vi "231124_Nikon_Led.vi"(8 "error in":errorcluster, 10 "Light path":u16(ring) items=["1- Eyepiece"=1, "2- Right"=2, "3- Left + Eyepiece"=3, "4- Left"=4], 11 "Microscope IN":T1={"Init"=FALSE, "ON / OFF"=FALSE, "Intensity"=102.0, "Objective"=2, "Light path"=1, "Z pos (µm)"=48440, "Eyepiece"=FALSE, "Right"=FALSE, "Left + Eyepiece"=FALSE, "Left"=FALSE} {"Z pos (µm)" min=0 max=990000 step=100 scale=0.0..990000.0; "Light path" items=["1- Eyepiece"=1, "2- Right"=2, "3- Left + Eyepiece"=3, "4- Left"=4]; "Objective" items=["1- Target"=1, "2- PLAN APO 100X 1,45 Oil"=2, "3- Empty"=3, "4- Empty"=4, "5- Empty"=5, "6- Empty"=6]; "Intensity" scale=0.0..2100.0}) -> (0 "error out":errorcluster, 3 "Microscope OUT":T1={"Init"=FALSE, "ON / OFF"=FALSE, "Intensity"=102.0, "Objective"=2, "Light path"=1, "Z pos (µm)"=48440, "Eyepiece"=FALSE, "Right"=FALSE, "Left + Eyepiece"=FALSE, "Left"=FALSE} {"Z pos (µm)" min=0 max=990000 step=100 scale=0.0..990000.0; "Light path" items=["1- Eyepiece"=1, "2- Right"=2, "3- Left + Eyepiece"=3, "4- Left"=4]; "Objective" items=["1- Target"=1, "2- PLAN APO 100X 1,45 Oil"=2, "3- Empty"=3, "4- Empty"=4, "5- Empty"=5, "6- Empty"=6]; "Intensity" scale=0.0..2100.0})   [LabVIEW 2024]
doc: "Thi vi displays LEDs accordingly to the lightpath"
panel:
  # "White light"
  # "Objective"
  # "Light path"
  # "Z pos (µm)"
  # "White light"
  # "Objective"
  # "Light path"
  # "Z pos (µm)"
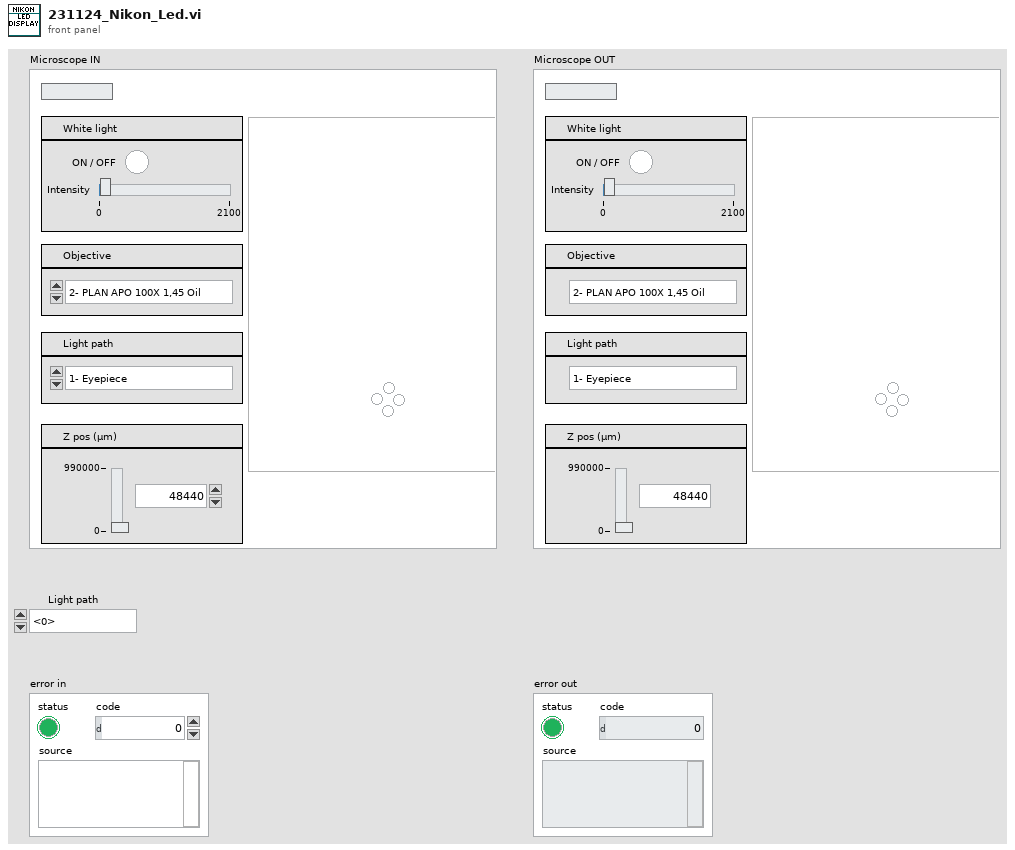
[diagram p1: front panel]
types:
  T1 = cluster{"Init":bool, "ON / OFF":bool, "Intensity":dbl, "Objective":i32, "Light path":u32, "Z pos (µm)":i32, "Eyepiece":bool, "Right":bool, "Left + Eyepiece":bool, "Left":bool}
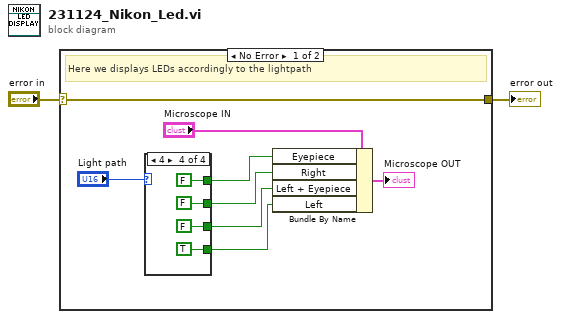
[diagram p0: block diagram]
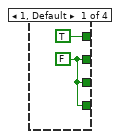
[diagram p2: hidden frame]
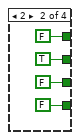
[diagram p3: hidden frame]
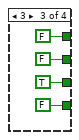
[diagram p4: hidden frame]
diagram:
  n1 = case shown="No Error" "error in" {
    selector: "error in" -> [w9 w25]
    tunnel: [w9 w25] -> w1
    frame No Error {
      # "Here we displays LEDs accordingly to the lightpath"
      n2 = case shown="4" "Light path" {
        tunnel: [TRUE FALSE FALSE FALSE] -> w8
        tunnel: [w11 TRUE FALSE FALSE] -> w7
        tunnel: [w11 FALSE TRUE FALSE] -> w6
        tunnel: [w11 FALSE FALSE TRUE] -> w5
        frame 1, Default {
          w11 = FALSE
        }
        frame 2 {
        }
        frame 3 {
        }
        frame 4 {
        }
      }
      n3 = Bundle By Name(cluster="Microscope IN", "Eyepiece"=w8, "Right"=w7, "Left + Eyepiece"=w6, "Left"=w5) -> (→"Microscope OUT":T1)
    }
    frame Error {
    }
  }
  "error out" <- w1
